vi "Read plots.vi"(9 "WaveformChart in":refnum<class "WaveformChart.lvclass">) -> (3 "WaveformChart out":refnum<class "WaveformChart.lvclass">, 4 "plots":refnum<class "Plot.lvclass">[](array[class]))   [LabVIEW 2014, in "Raspberry Pi Compatible Compiler for LabVIEW.lvlib" / "WaveformChart.lvclass"]
uses:
  WaveformChart.lvclass
  Plot/Plot.lvclass
  WaveformChart.lvclass/WaveformChart.ctl
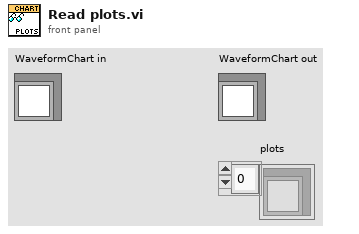
[diagram p1: front panel]
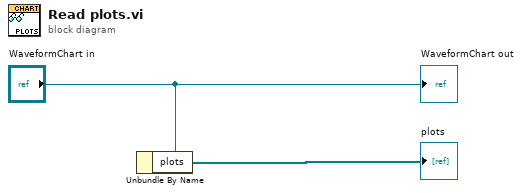
[diagram p0: block diagram]
diagram:
  n1 = Unbundle By Name("WaveformChart in") -> ("plots"=→"plots":refnum<class "Plot.lvclass">[])
  "WaveformChart out" <- "WaveformChart in"
